vi "_log_segmented_read.vi"(4 "Force binary format (T)":bool=TRUE, 5 "Total Segments":i32=1, 6 "Last Segment":bool=TRUE, 7 "Data":string, 8 "error in":errorcluster caption="error in (no error)", 9 "Previous Start Time ms":u32, 10 "Segment Ix":i32, 11 "VISA resource name":refnum<visa-resource-name>) -> (0 "error out":errorcluster, 1 "New Start Time ms":u32, 3 "VISA resource name out":refnum<visa-resource-name>)   [LabVIEW 2020, in "Rohde&Schwarz RTx Oscilloscopes.lvlib" / "rsidr_core.lvlib"]
uses:
  rsidr_core.lvlib
  type_Error_Codes.ctl
panel:
  out "First Start Time":u32
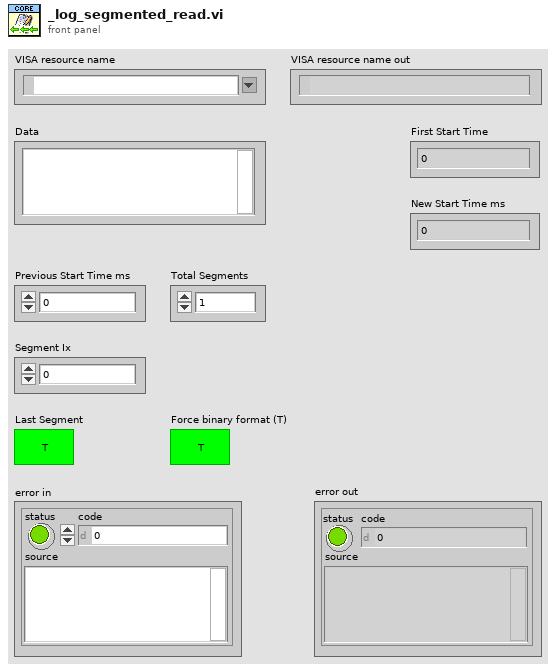
[diagram p1: front panel]
types:
  T1 = typedef "Rohde&Schwarz RTx Oscilloscopes.lvlib/rsidr_core.lvlib/type_Error_Codes.ctl" = enum16{"No_error", "VISA_err_ResourceNotFound", "VISA_err_Timeout", "VISA_warn_MoreDataAvailable", "RS_err_MissingCallback", "RS_err_InvalidAttribute", "RS_err_InvalidValue", "RS_err_UnknownResource", "RS_err_AlreadyInitialized", "RS_err_InstrumentStatus", "RS_err_BadRepCapName", "RS_err_TypesMismatch", "RS_err_ValueNotSupported", "RS_err_InvalidRngTable", "RS_err_IDqueryFail", "RS_err_UnexpResponse", "VISA_warn_ConfigNotLoaded", "RS_err_AttributeNotReadable", "RS_err_AttributeNotWritable", "RS_err_InstrumentType", "RS_err_InstrumentOption", "VISA_err_InvalidSize", "RS_err_ReliabilityIndicator", "VISA_warn_UnknownStatus", "VISA_warn_TermCharRead", "VISA_err_IO_error", "RS_err_FunctionNotSupported", "VISA_warn_QueueEmpty"}
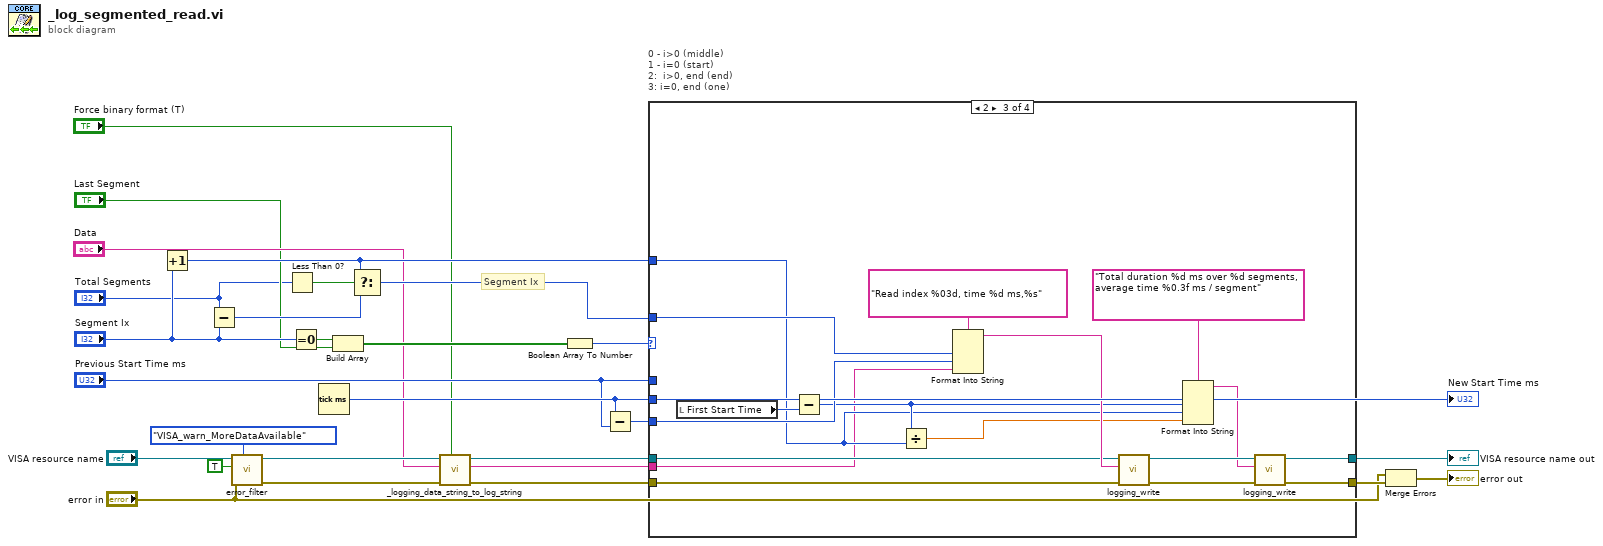
[diagram p0: block diagram]
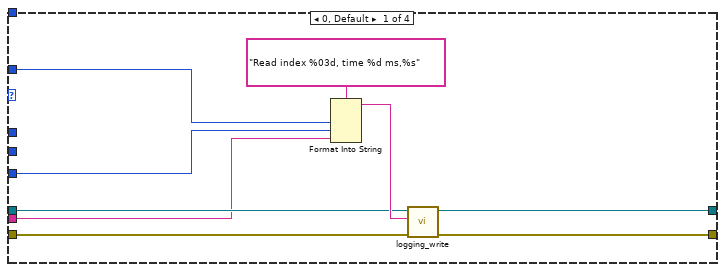
[diagram p2: hidden frame]
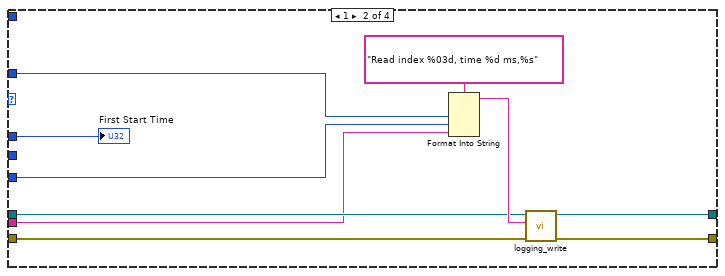
[diagram p3: hidden frame]
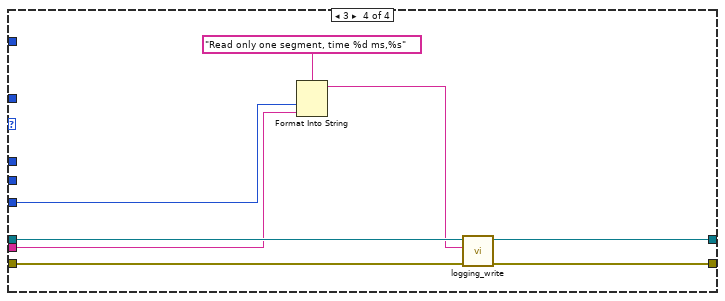
[diagram p4: hidden frame]
diagram:
  # "Segment Ix"
  n1 = Increment(x="Segment Ix") -> (x+1=w11:i32)
  n2 = Subtract(x="Total Segments", y="Segment Ix") -> (x-y=w14:i32)
  n3 = call "error_filter.vi"("Error Enum in"=type_Error_Codes."VISA_warn_MoreDataAvailable" ("Code to detect"), "error in"="error in", "Clear detected code (F)"=TRUE ("Clear detected error (F)"), "VISA resource name"="VISA resource name") -> ("error out"=w10:errorcluster, "VISA resource name out"=w9:refnum<visa-resource-name>)  [unwired: 5 in, 1 out]
  n4 = Less Than 0?(x="Total Segments") -> (x < 0?=w1:bool)
  n5 = Equal To 0?(x="Segment Ix") -> (x = 0?=w27:bool)
  n6 = Tick Count (ms)() -> (millisecond timer value=w22:u32)
  "New Start Time ms" <- w22
  n7 = Build Array(w27, "Last Segment") -> (w26:bool[])
  n8 = Select(t=w11, s=w1, f=w14) -> (s? t:f=w12:i32)
  n9 = call "_logging_data_string_to_log_string.vi"("Force binary format (F)"="Force binary format (T)", "error in"=w10, "Raw string to log"="Data", "VISA resource name"=w9) -> ("error out"=w8:errorcluster, "Result log string"=w5:string, "VISA resource name out"=w7:refnum<visa-resource-name>)  [unwired: 5 in]
  n10 = Boolean Array To Number(Boolean array=w26) -> (number=w25:u32)
  n11 = Subtract(x=w22, y="Previous Start Time ms") -> (x-y=w23:u32)
  n12 = case "0 - i>0 (middle)\n1 - i=0 (start)\n2:  i>0, end (end)\n3: i=0, end (one)" shown="2" w25 {
    tunnel: w8 -> [w34 w44 w62 w72]
    tunnel: w7 -> [w33 w43 w61 w71]
    tunnel: [w32 w42 w59 w68] -> w17
    tunnel: [w31 w41 w58 w67] -> w24
    tunnel: w23 -> [w30 w39 w60 w66]
    tunnel: "Previous Start Time ms" -> [_ w40 _ _]
    tunnel: w22 -> [_ _ w54 _]
    tunnel: w12 -> [w29 w38 w51 _]
    tunnel: w11 -> [_ _ w48 _]
    tunnel: w5 -> [w28 w37 w47 w65]
    frame 0, Default {
      n13 = Format Into String(format string="Read index %03d, time %d ms,%s", w29, w30, w28) -> (resulting string=w35:string)  [unwired: 2 in, 1 out]
      n14 = call "logging_write.vi"("error in"=w34, "String to write"=w35, "VISA resource name"=w33) -> ("error out"=w32:errorcluster, "VISA resource name out"=w31:refnum<visa-resource-name>)  [unwired: 7 in]
    }
    frame 1 {
      n15 = Format Into String(format string="Read index %03d, time %d ms,%s", w38, w39, w37) -> (resulting string=w45:string)  [unwired: 2 in, 1 out]
      n16 = call "logging_write.vi"("error in"=w44, "String to write"=w45, "VISA resource name"=w43) -> ("error out"=w42:errorcluster, "VISA resource name out"=w41:refnum<visa-resource-name>)  [unwired: 7 in]
      "First Start Time" <- w40
    }
    frame 2 {
      n17 = local read "First Start Time"() -> (w53:u32)
      n18 = Subtract(x=w54, y=w53) -> (x-y=w50:u32)
      n19 = Divide(x=w50, y=w48) -> (x/y=w49:dbl)
      n20 = Format Into String(format string="Read index %03d, time %d ms,%s", w51, w60, w47) -> (resulting string=w63:string)  [unwired: 2 in, 1 out]
      n21 = call "logging_write.vi"("error in"=w62, "String to write"=w63, "VISA resource name"=w61) -> ("error out"=w57:errorcluster, "VISA resource name out"=w56:refnum<visa-resource-name>)  [unwired: 7 in]
      n22 = Format Into String(format string="Total duration %d ms over %d segments, average time %0.3f ms / segment", w50, w48, w49) -> (resulting string=w52:string)  [unwired: 2 in, 1 out]
      n23 = call "logging_write.vi"("error in"=w57, "String to write"=w52, "VISA resource name"=w56) -> ("error out"=w59:errorcluster, "VISA resource name out"=w58:refnum<visa-resource-name>)  [unwired: 7 in]
    }
    frame 3 {
      n24 = Format Into String(format string="Read only one segment, time %d ms,%s", w66, w65) -> (resulting string=w69:string)  [unwired: 2 in, 1 out]
      n25 = call "logging_write.vi"("error in"=w72, "String to write"=w69, "VISA resource name"=w71) -> ("error out"=w68:errorcluster, "VISA resource name out"=w67:refnum<visa-resource-name>)  [unwired: 7 in]
    }
  }
  "VISA resource name out" <- w24
  n26 = Merge Errors("error in", w17) -> (→"error out":errorcluster)
